vi "UDP Multicast Open.vi"   [LabVIEW 2017]
doc: "Opens a UDP multicast socket on the <B>port</B>. You must manually select the polymorphic instance you want to use."
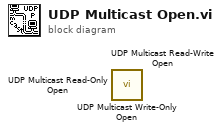
[diagram p0: block diagram]
diagram:
  n1 = call <vilib>:"UDP Multicast Write-Only Open.vi"() -> ()  [unwired: 10 in, 2 out]
  n2 = call <vilib>:"UDP Multicast Read-Write Open.vi"() -> ()  [unwired: 9 in, 3 out]
  n3 = call <vilib>:"UDP Multicast Read-Only Open.vi"() -> ()  [unwired: 9 in, 3 out]
